vi "Clock.vi"() -> ()   [LabVIEW 2020]
uses:
  <vilib>/numeric/Random Number (Range).vi
  <vilib>/numeric/Random Number (Range) U64.vi
  Fire/Spread Fire.vi
  <vilib>/numeric/sub_Random U32.vi
panel:
  in  "Snooze":bool
  out "Clock Fire":i32[][](graph)
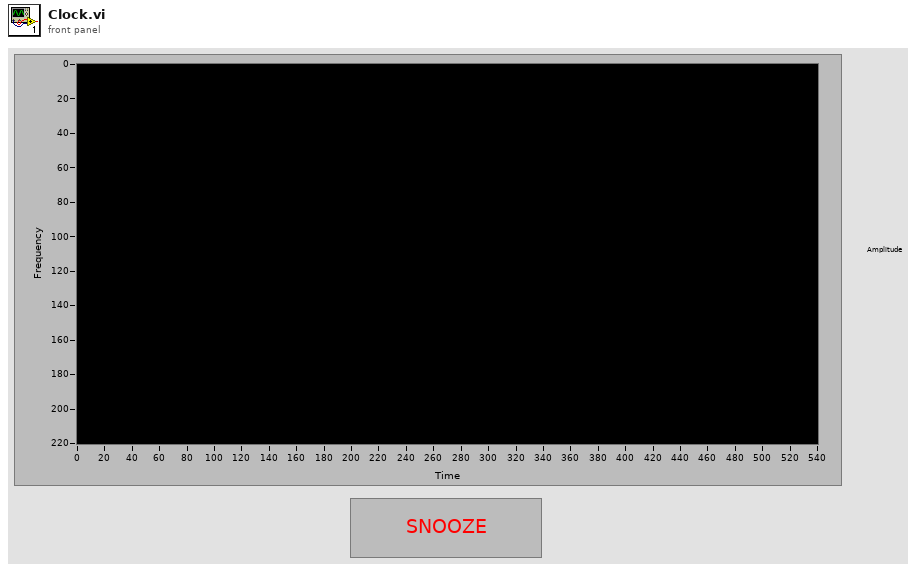
[diagram p1: front panel]
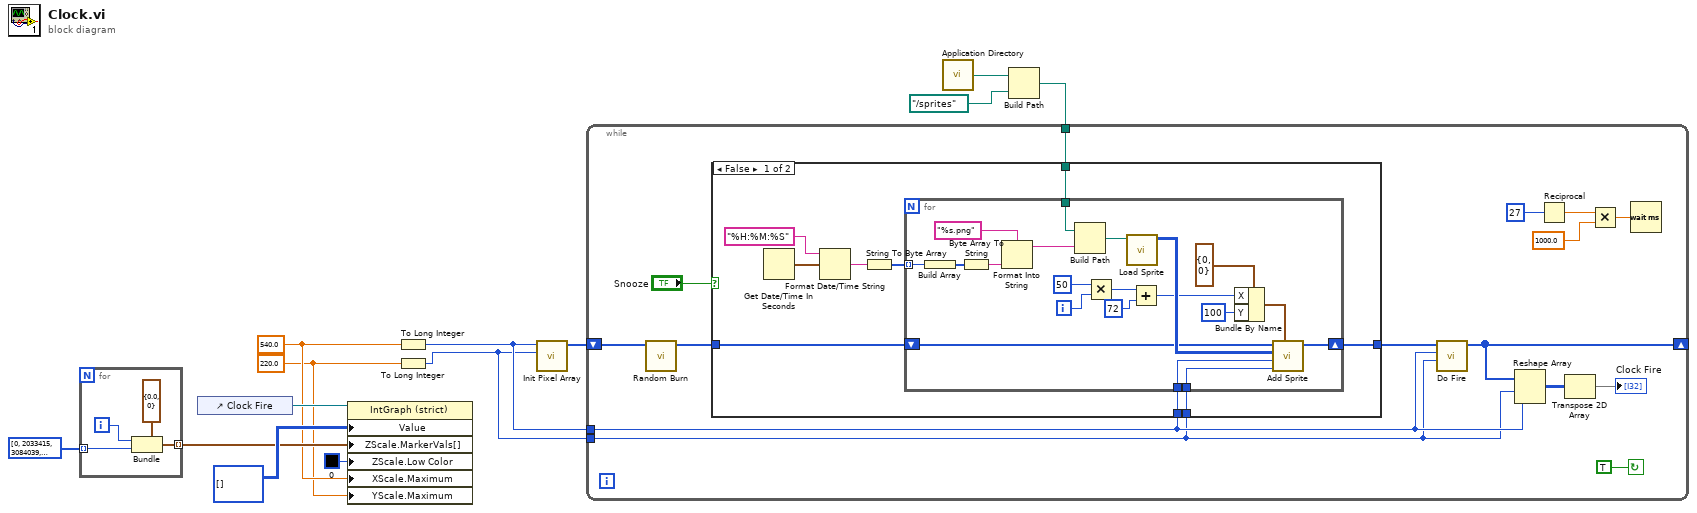
[diagram p0: block diagram]
diagram:
  w7 = 220.0 ("X Scale.Range:Maximum")
  w8 = 540.0 ("X Scale.Range:Maximum")
  n1 = for {
    tunnel: u32[] [0, 2033415, 3084039, 4656903, 5707527, 6758151, 7806727, 9381639, 10432263, 11484935, 12535559, 13059847, 14634759, 14636807, 14636807, 14114567, 14114567, 14116623, 13594383, 13596431, 13598479, 13600535, 13076247, 13078295, 13080351, 12558111, 12558111, 12560167, 12560167, 12562223, 12037935, 12039983, 12039991, 13619055, 14671775, 15724487, 16777215] ("Array") -> [w15] mode=indexing
    tunnel: [w14] -> w11 mode=indexing
    i -> [w16]
    n2 = Bundle(cluster=cluster{dbl, u32} {0.0, 0}, w16, w15) -> (w14:cluster{dbl, u32})
  }
  n3 = control-ref of="Clock Fire"() -> (w10:refnum<vi>)
  n4 = property class="IntGraph (strict)"(reference=w10, "Value"=i32[][] [] ("Hell Fire"), "ZScale.MarkerVals[]"=w11, "ZScale.Low Color"=u32 0 ("Z Scale.Low Color"), "XScale.Maximum"=w8, "YScale.Maximum"=w7) -> ()  [unwired: 1 in, 2 out]
  n5 = To Long Integer(number=w8) -> (32bit integer=w6:i32)
  n6 = To Long Integer(number=w7) -> (32bit integer=w5:i32)
  n7 = call "Init Pixel Array.vi"("Height"=w5, "Width"=w6) -> ("Pixel Array"=w4:i32[])  [unwired: 9 in]
  n8 = call <vilib>:"Application Directory.vi"() -> ("Application Directory"=w3:path)
  n9 = Build Path(base path=w3, name or relative path=path "../sprites" ("Path to PNG file")) -> (appended path=w1:path)
  n10 = while {
    shift-right: [w27] -> _
    shift-left: w4 -> [w25]
    tunnel: w6 -> [w23]
    tunnel: w5 -> [w22]
    tunnel: w1 -> [w21]
    stop <- TRUE continue-if-true
    n11 = call "Random Burn.vi"("Pixel Array In"=w25) -> ("Pixel Array Out"=w24:i32[])  [unwired: 10 in]
    n12 = case shown="False" "Snooze" {
      tunnel: w24 -> [w39 w62]
      tunnel: w23 -> [w38 _]
      tunnel: w22 -> [w37 _]
      tunnel: w21 -> [w36 _]
      tunnel: [w33 w62] -> w20
      frame False {
        n13 = Get Date/Time In Seconds() -> (seconds since 1Jan1904=w40:timestamp)
        n14 = Format Date/Time String(time format string (%c)="%H:%M:%S", seconds (now)=w40) -> (date/time string=w35:string)  [unwired: 1 in]
        n15 = String To Byte Array(string=w35) -> (unsigned byte array=w34:u8[])
        n16 = for {
          tunnel: w34 -> [w48] mode=indexing
          shift-right: [w59] -> w33
          shift-left: w39 -> [w60]
          tunnel: w38 -> [w58]
          tunnel: w37 -> [w57]
          tunnel: w36 -> [w53]
          i -> [w49]
          n17 = Build Array(w48) -> (w47:u8[])
          n18 = Byte Array To String(unsigned byte array=w47) -> (string=w46:string)
          n19 = Format Into String(format string="%s.png", w46) -> (resulting string=w50:string)  [unwired: 2 in, 1 out]
          n20 = Build Path(base path=w53, name or relative path=w50) -> (appended path=w52:path)
          n21 = Multiply(x=50, y=w49) -> (x*y=w45:i32)
          n22 = call "Load Sprite.vi"("Path to PNG file"=w52) -> ("Sprite Array"=w61:i32[][])  [unwired: 10 in]
          n23 = Add(x=w45, y=72) -> (x+y=w43:i32)
          n24 = Bundle By Name(cluster=cluster{"X":i16, "Y":i16} {"X"=0, "Y"=0} ("Point"), "X"=w43, "Y"=i16 100) -> (w55:cluster{"X":i16, "Y":i16})
          n25 = call "Add Sprite.vi"("Point"=w55, "Height"=w57, "Width"=w58, "Sprite Array In"=w61, "Pixel Array In"=w60) -> ("Pixel Array Out"=w59:i32[])  [unwired: 6 in]
        }
      }
      frame True {
      }
    }
    n26 = call "Do Fire.vi"("Height"=w22, "Width"=w23, "Pixel Array In"=w20) -> ("Pixel Array Out"=w27:i32[])  [unwired: 8 in]
    n27 = Reshape Array(w27, w22, w23) -> (w26:i32[][])
    n28 = Reciprocal(x=27 ("FPS")) -> (1/x=w31:dbl)
    n29 = Transpose 2D Array(2D array=w26) -> (transposed array=→"Clock Fire":i32[][])
    n30 = Multiply(x=w31, y=1000.0) -> (x*y=w29:dbl)
    n31 = Wait (ms)(milliseconds to wait=w29) -> ()  [unwired: 1 out]
  }
